vi "AVS_GetSaturatedPixels.vi"(0 "a_hDevice":i32, 7 "a_pSaturated":u8[](array[numeric])) -> (4 "Output Value":i32, 8 "a_pSaturated":u8[](array[numeric]))   [LabVIEW 2016]
uses:
  libavs.so
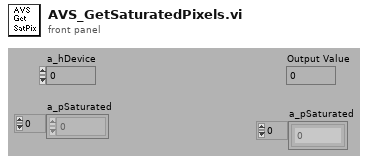
[diagram p1: front panel]
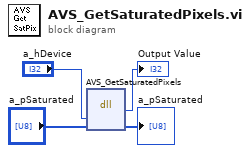
[diagram p0: block diagram]
diagram:
  n1 = dll-call lib="home/harini/tcs/ts_sedspectrometer/ss_sedspectrometer/VIs/libavs.so" fn="AVS_GetSaturatedPixels"("a_hDevice"="a_hDevice", "a_pSaturated"="a_pSaturated") -> ("return type"=→"Output Value":i32, "a_pSaturated"=→"a_pSaturated":u8[])  [unwired: 4 in, 2 out]
